vi "SerialNumber.vi"() -> ()   [LabVIEW 2013]
panel:
  in  "SerialNumber":string
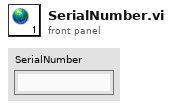
[diagram p1: front panel]
diagram:
